vi "Creep Mode.vi"(8 "Throttle In":dbl, 10 "Steer In":dbl, 11 "D-Pad":T1) -> (0 "Throttle Out":dbl, 2 "Steer Out":dbl)   [LabVIEW 2014]
uses:
  Real-Life Controls/D-Pad.ctl
  Robot Global Data.vi
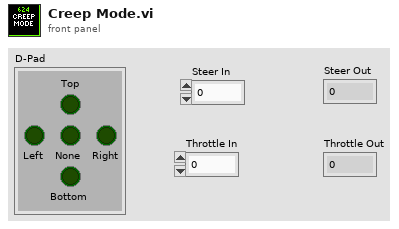
[diagram p1: front panel]
types:
  T1 = typedef "D-Pad.ctl" = cluster{"Top":bool, "Bottom":bool, "None":bool, "Right":bool, "Left":bool}
  T2 = typedef "Dashboard Control Data.ctl" = cluster{"Cam Exposure":dbl, "Go to angle":dbl, "Steer PID Gains":cluster{"proportional gain (Kc)":dbl, "integral time (Ti, min)":dbl, "derivative time (Td, min)":dbl}, "Steer PID output Range":cluster{"output high":dbl, "output low":dbl}, "Pressure m \nValue":dbl, "Pressure b \nValue":dbl, "Roller Command Cluster ":T3, "Elevator":T4, "Encoder Control":T6, "Auton Settings":cluster{"Drive Dist Window Size":dbl}, "Drivetrain Settings":T7, "Pike":T8}
  T3 = typedef "Roller Control.ctl" = cluster{"Intake Speed":dbl, "Turn In Speed":dbl, "Unload Speed":dbl, "Turn Out Speed":dbl, "Ping Align Tolerance":dbl, "Tote Range Threshold":dbl, "Right Pot 0":dbl, "Pot Threshold":dbl, "Left Pot 0":dbl, "Manual 0s?":bool, "Right Pot Scale":dbl, "Left Pot Scale":dbl, "0 wait time":i32, "Zero Pots":bool, "Min Elevator Height":dbl, "Eject Time":dbl, "Eject US Threshold":dbl, "Anti-Twitch Time":u32, "Ping Caring Threshold":dbl, "Pot Diff Threshold":dbl, "Pinch Sustain":u32, "Absorb Give Up Threshold":dbl, "Untip In Threshold":dbl, "Untip Grab Range":dbl, "Ultrasonic Hold Time":u32, "Landscape Absorb Time":u32, "Pot Use Wait Time":u32, "Can Turn Stop Range":dbl, "Ignore Pressure":bool, "HP Load Speed":dbl}
  T4 = typedef "Elevator DB Control.ctl" = cluster{"PID Output Range":cluster{"output high":dbl, "output low":dbl}, "PID gains":cluster{"proportional gain (Kc)":dbl, "integral time (Ti, min)":dbl, "derivative time (Td, min)":dbl}, "Height Tolerance":sgl, " Encoder Constant":dbl, "Safe Mode Max Speed":sgl, "Eject Time":sgl, "Zeroing Speed":sgl, "Presets":T5, "Ping Detect Threshold":sgl, "Trashcan Detect Threshold":sgl, "Zero Filter Time":dbl, "Stabilizer Open Time":dbl, "Zero Creep Speed":dbl, "Max Current":dbl, "Current Trip Time":dbl, "Abort Pitch":dbl, "Finger m":dbl, "Finger b":dbl, "Finger max ":dbl, "Finger Stabilizer":dbl, "Finger Store":dbl, "Finger Stop Store":dbl, "Stabilizer Close Time":dbl, "HP Finger Store":dbl, "HP Finger Stop Store":dbl, "Finger min":dbl, "Unstick gain":dbl, "Roller Wait":dbl}
  T5 = typedef "Elevator Presets.ctl" = cluster{"Pickup 2 w/ Tote":sgl, "Pickup 2 w/ Trashcan":sgl, "Pickup 3 w/ Tote":sgl, "Pickup 3 w/ Trashcan":sgl, "Bottom":sgl, "Pickup 1 w/ Tote":sgl, "Pickup Trashcan":sgl, "Pickup 1 w/ Trashcan":sgl, "Eject":sgl, "Hold Low":sgl, "Step add height":sgl, "Untip Lift":dbl, "Drop Stack":dbl, "HP Load Hold":dbl, "HP Load Drop":dbl, "HP Load Finger":dbl, "HP Load Hold Can":dbl, "Store can max":dbl, "HP Drag Score":dbl, "HP Store can max":dbl, "HP Drag Finish":dbl, "HP Carry min":dbl, "HP Finger Anti-Crash":dbl, "Finger trashcan avoid":dbl}
  T6 = typedef "Encoder Control.ctl" = cluster{"Left Tick Constant":dbl, "Right Tick Constant":dbl, "Center Tick Constant":dbl, "Reset?":bool, "Y Dist":cluster{"PID gains":cluster{"proportional gain (Kc)":dbl, "integral time (Ti, min)":dbl, "derivative time (Td, min)":dbl}}, "X Dist":cluster{"PID gains":cluster{"proportional gain (Kc)":dbl, "integral time (Ti, min)":dbl, "derivative time (Td, min)":dbl}}, "Y Stop Thresh":dbl, "Y Stop Speed":dbl, "X Stop Thresh":dbl, "X Stop Speed":dbl}
  T7 = typedef "Drivetrain Settings.ctl" = cluster{"Gyro Tolerance":sgl, "Strafe Correct max steer":sgl, "Strafe Timer Wait":sgl, "Throttle Ramp (ms)":sgl, "Strafe Ramp (ms)":sgl, "Angular rate compensation":bool, "Throttle to Rate Scale":sgl, "Rate compensation gain":sgl, "Creep Steer":sgl, "Creep Throttle":sgl}
  T8 = typedef "Pike DB Controls.ctl" = cluster{"Down Speed":dbl, "Up Speed":dbl, "Max Down Time":dbl, "Max Up Time":dbl, "Current Limit":dbl}
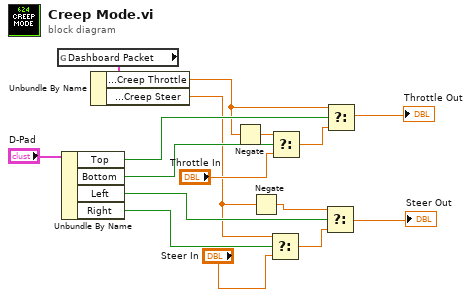
[diagram p0: block diagram]
diagram:
  n1 = global read "Robot Global Data.vi" "Dashboard Packet"() -> (w5:T2)
  n2 = Unbundle By Name("D-Pad") -> ("Top"=w8:bool, "Bottom"=w7:bool, "Left"=w14:bool, "Right"=w15:bool)
  n3 = Unbundle By Name(w5) -> ("Drivetrain Settings.Creep Throttle"=w3:sgl, "Drivetrain Settings.Creep Steer"=w1:sgl)
  n4 = Negate(x=w3) -> (-x=w4:sgl)
  n5 = Negate(x=w1) -> (-x=w2:sgl)
  n6 = Select(t=w1, s=w15, f="Steer In") -> (s? t:f=w12:dbl)
  n7 = Select(t=w4, s=w7, f="Throttle In") -> (s? t:f=w10:dbl)
  n8 = Select(t=w2, s=w14, f=w12) -> (s? t:f=→"Steer Out":dbl)
  n9 = Select(t=w3, s=w8, f=w10) -> (s? t:f=→"Throttle Out":dbl)
